vi "OlympusTest.vi"(8 "error in (no error)":errorcluster, 10 "String":string, 11 "Instrument Port":refnum<visa-resource-name>="IX2-UCB") -> (0 "error out":errorcluster, 3 "Result":string)   [LabVIEW 2018, in "Olympus IX BX Series.lvlib"]
uses:
  Olympus IX BX Series.lvlib
panel:
  in  "Device Number\n(1: -Condensor\n     - Objective\n     - Lamp\n     - Shutter\n2: - Z-Motion\n   - Autofocus)":i32=1
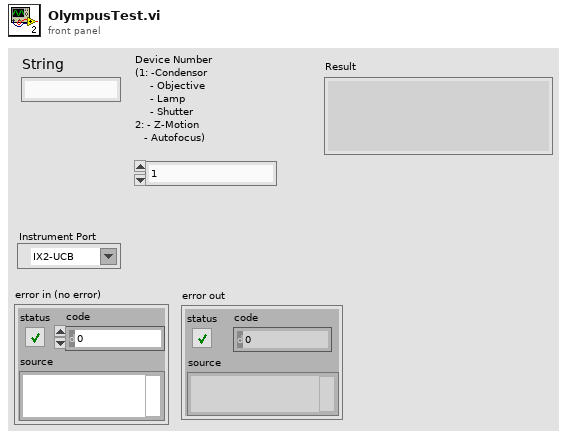
[diagram p1: front panel]
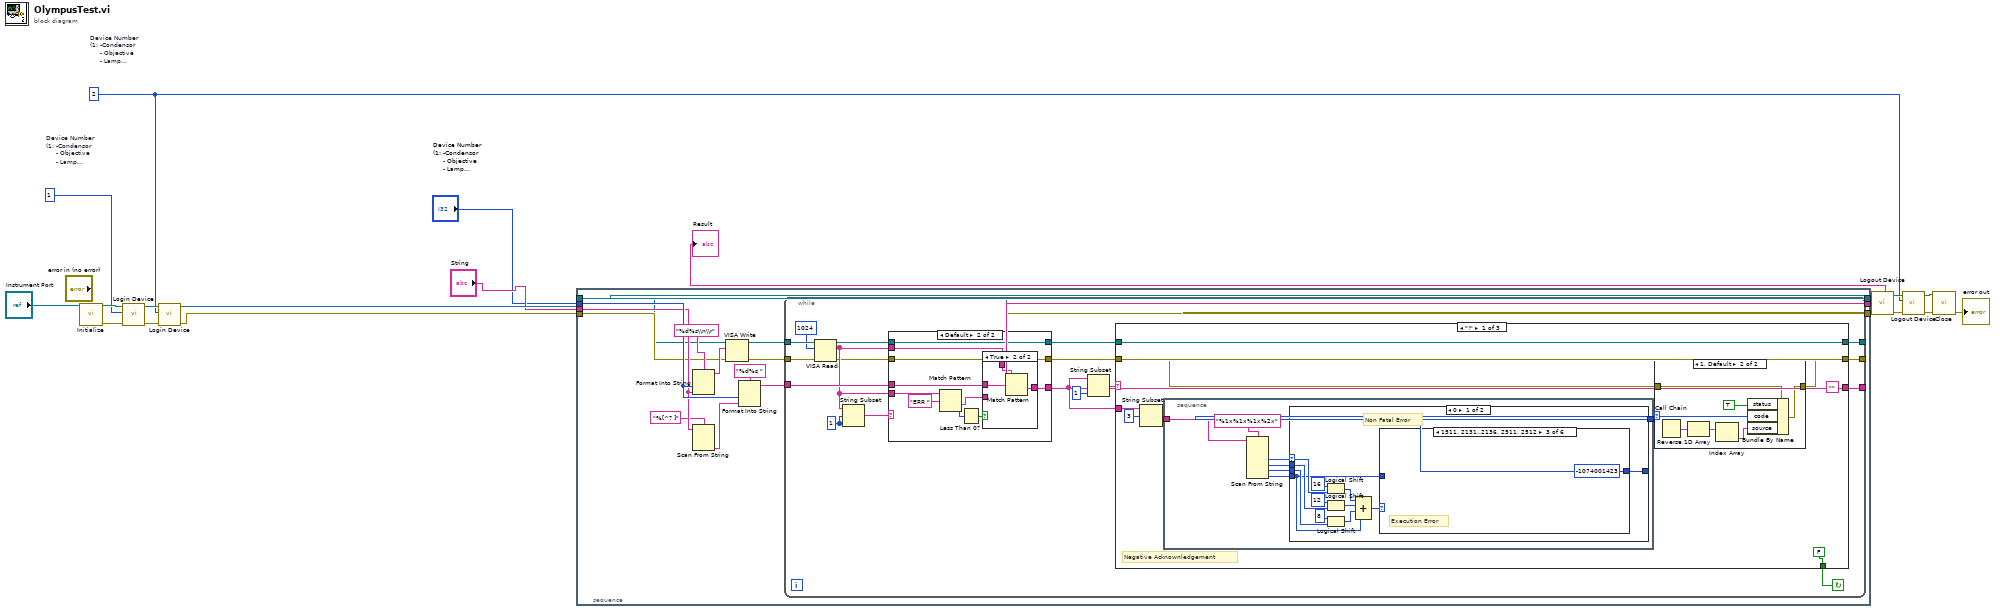
[diagram p0: block diagram]
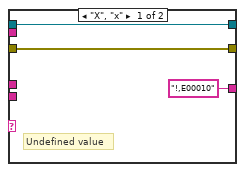
[diagram p2: hidden frame]
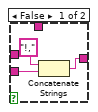
[diagram p3: hidden frame]
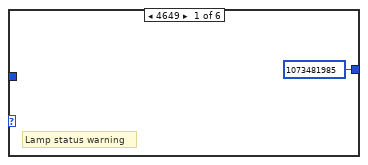
[diagram p4: hidden frame]
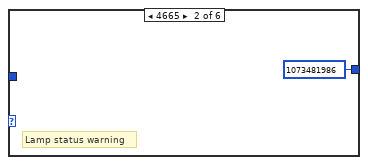
[diagram p5: hidden frame]
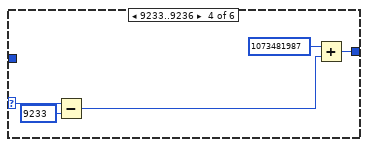
[diagram p6: hidden frame]
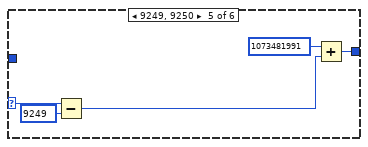
[diagram p7: hidden frame]
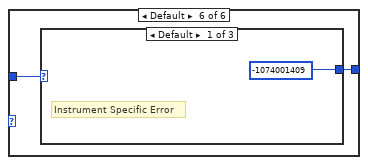
[diagram p8: hidden frame]
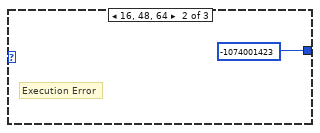
[diagram p9: hidden frame]
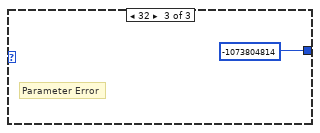
[diagram p10: hidden frame]
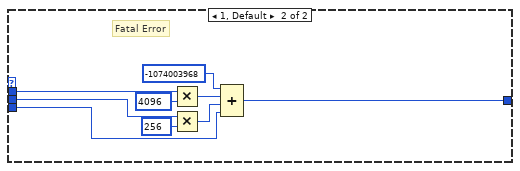
[diagram p11: hidden frame]
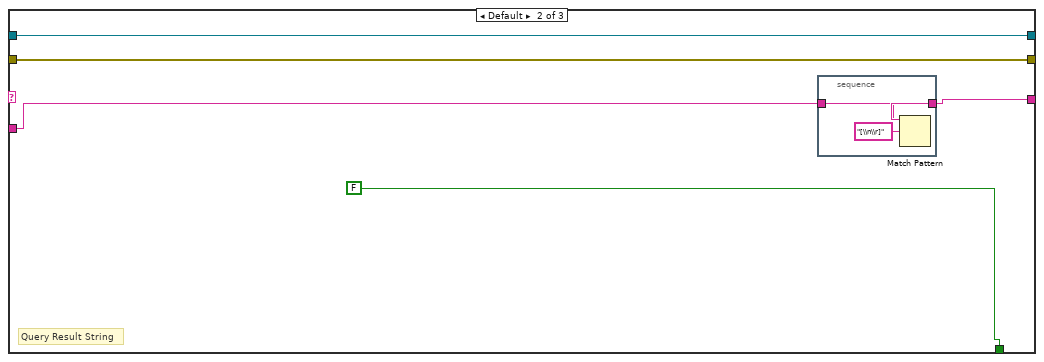
[diagram p13: hidden frame]
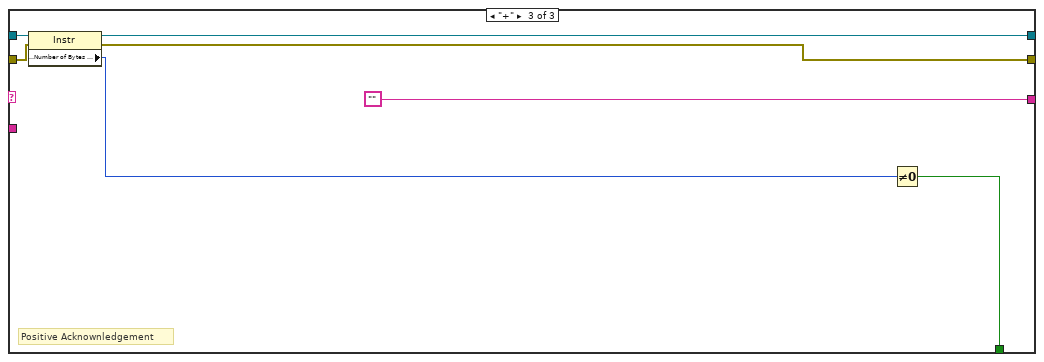
[diagram p14: hidden frame]
diagram:
  w9 = 2  # Device Number (1: -Condensor      - Objective      - Lamp      - Shutter 2: - Z-Motion    - Autofocus)
  w3 = 1  # Device Number (1: -Condensor      - Objective      - Lamp      - Shutter 2: - Z-Motion    - Autofocus)
  n1 = call "Initialize.vi"("VISA Resource Name"="Instrument Port") -> ("VISA Resource Name Out"=w17:refnum<visa-resource-name>, "error out"=w16:errorcluster)  [unwired: 13 in]
  n2 = call "Login Device.vi"("error in (no error)"=w16, "Device Number (1)"=w3, "VISA Resource Name"=w17) -> ("error out"=w14:errorcluster, "VISA Resource Name Out"=w15:refnum<visa-resource-name>)  [unwired: 7 in]
  n3 = call "Login Device.vi"("error in (no error)"=w14, "Device Number (1)"=w9, "VISA Resource Name"=w15) -> ("error out"=w7:errorcluster, "VISA Resource Name Out"=w8:refnum<visa-resource-name>)  [unwired: 7 in]
  n4 = stacked-sequence {
    tunnel: [w32] -> w5
    tunnel: [w34] -> w4
    tunnel: [w33] -> w6
    tunnel: w7 -> [w21]
    tunnel: "String" -> [w27]
    tunnel: "Device Number\n(1: -Condensor\n     - Objective\n     - Lamp\n     - Shutter\n2: - Z-Motion\n   - Autofocus)" -> [w28]
    tunnel: w8 -> [w20]
    frame #0 {
      n5 = Format Into String(format string="%d%s\\n\\r", w28, w27) -> (resulting string=w26:string)  [unwired: 2 in, 1 out]
      n6 = Scan From String(format string="%[^? ]", input string=w27) -> (output 1=w29:string)  [unwired: 3 in, 3 out]
      n7 = VISA Write(VISA resource name=w20, write buffer=w26, error in (no error)=w21) -> (VISA resource name out=w24:refnum<visa-resource-name>, error out=w23:errorcluster)  [unwired: 1 out]
      n8 = Format Into String(format string="%d%s ", w28, w29) -> (resulting string=w31:string)  [unwired: 2 in, 1 out]
      n9 = while {
        tunnel: w23 -> [w52]
        tunnel: w24 -> [w51]
        tunnel: w31 -> [w49]
        tunnel: [w48] -> w32
        tunnel: [w47] -> w33
        tunnel: [w46] -> w34
        stop <- w42 continue-if-true
        w41 = 1 ("length (rest)")
        n10 = VISA Read(VISA resource name=w51, byte count=u32 1024, error in (no error)=w52) -> (VISA resource name out=w38:refnum<visa-resource-name>, read buffer=w39:string, error out=w36:errorcluster)  [unwired: 1 out]
        n11 = String Subset(string=w39, offset (0)=w41, length (rest)=w41) -> (substring=w40:string)
        n12 = case shown="Default" w40 {
          tunnel: w49 -> [_ w65]
          tunnel: ["!,E00010" w64] -> w45
          tunnel: w39 -> [_ w59]
          tunnel: w39 -> [_ w58]
          tunnel: w38 -> [w55 w57]
          tunnel: [w55 w57] -> w37
          tunnel: w36 -> [w54 w56]
          tunnel: [w54 w56] -> w35
          frame "X", "x" {
            # "Undefined value"
          }
          frame Default {
            n13 = Match Pattern(string=w58, regular expression="ERR ") -> (after substring=w60:string, offset past match=w62:i32)  [unwired: 1 in, 2 out]
            n14 = Less Than 0?(x=w62) -> (x < 0?=w61:bool)
            n15 = case shown="True" w61 {
              tunnel: w65 -> [_ w71]
              tunnel: [w67 w70] -> w64
              tunnel: w59 -> [_ w69]
              tunnel: w60 -> [w68 _]
              frame False {
                n16 = Concatenate Strings("!," ("string"), w68) -> (w67:string)
              }
              frame True {
                n17 = Match Pattern(string=w69, regular expression=w71) -> (after substring=w70:string)  [unwired: 1 in, 3 out]
              }
            }
          }
        }
        n18 = String Subset(string=w45, length (rest)=1 ("length (rest)")) -> (substring=w44:string)  [unwired: 1 in]
        n19 = case shown="\"!\"" w44 {
          tunnel: w35 -> [w74 w139 w147]
          tunnel: [w73 w139 w145] -> w48
          tunnel: w35 -> [_ _ _]
          tunnel: [w79 w138 w146] -> w47
          tunnel: w37 -> [w79 w138 w148]
          tunnel: ["" w136 ""] -> w46
          tunnel: w45 -> [w78 w137 _]
          tunnel: [FALSE FALSE w143] -> w42
          frame "!" {
            # "Negative Acknownledgement"
            n20 = String Subset(string=w78, offset (0)=3) -> (substring=w76:string)  [unwired: 1 in]
            n21 = stacked-sequence {
              tunnel: [w87] -> w75
              tunnel: w76 -> [w82]
              frame #0 {
                n22 = Scan From String(format string="%1x%1x%1x%2x", input string=w82) -> (output 1=w83:u32, output 2=w84:u32, output 3=w85:u32, output 4=w86:u32)  [unwired: 6 in, 3 out]
                n23 = case shown="0" w83 {
                  selector: w83 -> [w97 _]
                  tunnel: w84 -> [w96 w125]
                  tunnel: w85 -> [w95 w124]
                  tunnel: w86 -> [w89 w119]
                  tunnel: [w99 w118] -> w87
                  frame 0 {
                    # "Non Fatal Error"
                    n24 = Logical Shift(y=16, x=w97) -> (x << y=w92:u32)
                    n25 = Logical Shift(y=12, x=w96) -> (x << y=w91:u32)
                    n26 = Logical Shift(y=8, x=w95) -> (x << y=w90:u32)
                    n27 = Compound Arithmetic op=ADD(w92, w91, w90, w89) -> (w88:u32)
                    n28 = case shown="1511, 2131..2136, 2511, 2512" w88 {
                      selector: w88 -> [_ _ _ w107 w112 _]
                      tunnel: [1073481985 1073481986 -1074001423 w105 w110 w114] -> w99
                      tunnel: w89 -> [_ _ _ _ _ w113]
                      frame 4649 {
                        # "Lamp status warning"
                      }
                      frame 4665 {
                        # "Lamp status warning"
                      }
                      frame 5393, 8497..8502, 9489, 9490 {
                        # "Execution Error"
                      }
                      frame 9233..9236 {
                        n29 = Subtract(x=w107, y=9233) -> (x-y=w103:u32)
                        n30 = Add(x=1073481987, y=w103) -> (x+y=w105:u32)
                      }
                      frame 9249, 9250 {
                        n31 = Subtract(x=w112, y=9249) -> (x-y=w108:u32)
                        n32 = Add(x=1073481991, y=w108) -> (x+y=w110:u32)
                      }
                      frame Default {
                        n33 = case shown="Default" w113 {
                          tunnel: [-1074001409 -1074001423 -1073804814] -> w114
                          frame Default {
                            # "Instrument Specific Error"
                          }
                          frame 16, 48, 64 {
                            # "Execution Error"
                          }
                          frame 32 {
                            # "Parameter Error"
                          }
                        }
                      }
                    }
                  }
                  frame 1, Default {
                    # "Fatal Error"
                    n34 = Multiply(x=w125, y=4096) -> (x*y=w121:u32)
                    n35 = Multiply(x=w124, y=256) -> (x*y=w120:u32)
                    n36 = Compound Arithmetic op=ADD(-1074003968, w121, w120, w119) -> (w118:u32)
                  }
                }
              }
            }
            n37 = case shown="1, Default" w75 {
              selector: w75 -> [_ w131]
              tunnel: w74 -> [w127 w132]
              tunnel: [w127 w128] -> w73
              frame 0 {
              }
              frame 1, Default {
                n38 = Call Chain() -> (call chain=w134:string[])
                n39 = Reverse 1D Array(array=w134) -> (reversed array=w133:string[])
                n40 = Index Array(array=w133) -> (element=w130:string)  [unwired: 1 in]
                n41 = Bundle By Name(cluster=w132, "status"=TRUE, "code"=w131, "source"=w130) -> (w128:errorcluster)
              }
            }
          }
          frame Default {
            # "Query Result String"
            n42 = stacked-sequence {
              tunnel: [w142] -> w136
              tunnel: w137 -> [w140]
              frame #0 {
                n43 = Match Pattern(string=w140, regular expression="[\\n\\r]") -> (before substring=w142:string)  [unwired: 1 in, 3 out]
              }
            }
          }
          frame "+" {
            # "Positive Acknownledgement"
            n44 = property class="Instr"(reference=w148, error in=w147) -> (reference out=w146:refnum<visa-resource-name>, error out=w145:errorcluster, "Serial Settings:Number of Bytes at Serial Port"=w144:u32)
            n45 = Not Equal To 0?(x=w144) -> (x != 0?=w143:bool)
          }
        }
      }
    }
  }
  "Result" <- w4
  n46 = call "Logout Device.vi"("error in (no error)"=w5, "VISA Resource Name"=w6) -> ("error out"=w12:errorcluster, "VISA Resource Name Out"=w13:refnum<visa-resource-name>)  [unwired: 8 in]
  n47 = call "Logout Device.vi"("error in (no error)"=w12, "Device Number (1)"=w9, "VISA Resource Name"=w13) -> ("error out"=w10:errorcluster, "VISA Resource Name Out"=w11:refnum<visa-resource-name>)  [unwired: 7 in]
  n48 = call "Close.vi"("VISA Resource Name"=w11, "error in (no error)"=w10) -> ("error out"=→"error out":errorcluster)  [unwired: 13 in]
